vi "ReadMessageAttribute.vi"(8 "error in":errorcluster, 10 "attribute name":string, 11 "message in":T1) -> (0 "error out":errorcluster, 1 "found?":bool, 2 "attribute":variant, 3 "message out":T1)   [LabVIEW 2013, in "CLM_LocalMessage.lvclass"]
uses:
  CLM_LocalMessage.lvclass
  Message.ctl
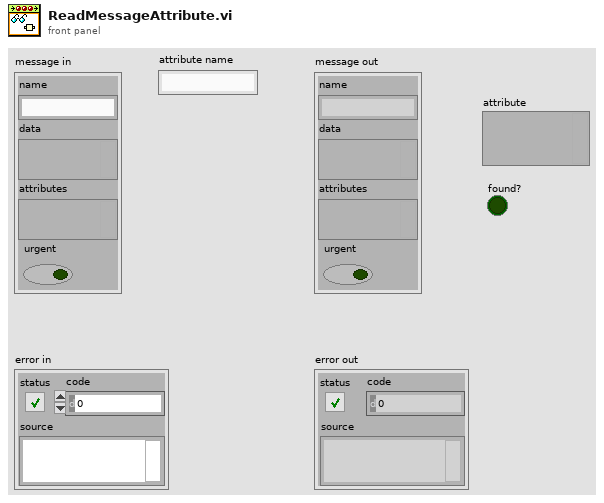
[diagram p1: front panel]
types:
  T1 = typedef "CLM_LocalMessage.lvclass/Message.ctl" = cluster{"name":string, "data":variant, "attributes":variant, "urgent":bool}
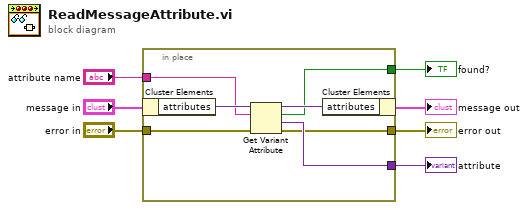
[diagram p0: block diagram]
diagram:
  n1 = in-place {
    in-place-border: "attribute name" -> [w13]
    in-place-border: [w11] -> w4
    in-place-border: [w10] -> w3
    in-place-border: "error in" -> [w9]
    in-place-border: [w8] -> w1
    n2 = in-place-cluster #1("message in") -> ("attributes"=w14:variant)
    n3 = Get Variant Attribute(Variant=w14, name=w13, error in=w9) -> (duplicate Variant=w12:variant, found=w11:bool, value=w10:variant, error out=w8:errorcluster)  [unwired: 1 in]
    n4 = in-place-cluster #1("attributes"=w12) -> (→"message out":T1)
  }
  "found?" <- w4
  "attribute" <- w3
  "error out" <- w1
